vi "CS_Write_Config.vi"(4 "error in (no error)":errorcluster, 7 "Config refnum":T1) -> (0 "error out":errorcluster, 3 "refnum out":T1)   [LabVIEW 2015]
uses:
  <vilib>/Utility/config.llb/Config Data RefNum.ctl
  GSP_Wavelength_Global.vi
  <vilib>/Utility/config.llb/Write Key (Double).vi
  <vilib>/Utility/config.llb/NI_LVConfig.lvlib
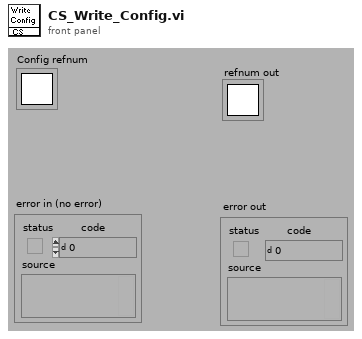
[diagram p1: front panel]
types:
  T1 = typedef "NI_LVConfig.lvlib/Config Data RefNum.ctl" = refnum<k1>
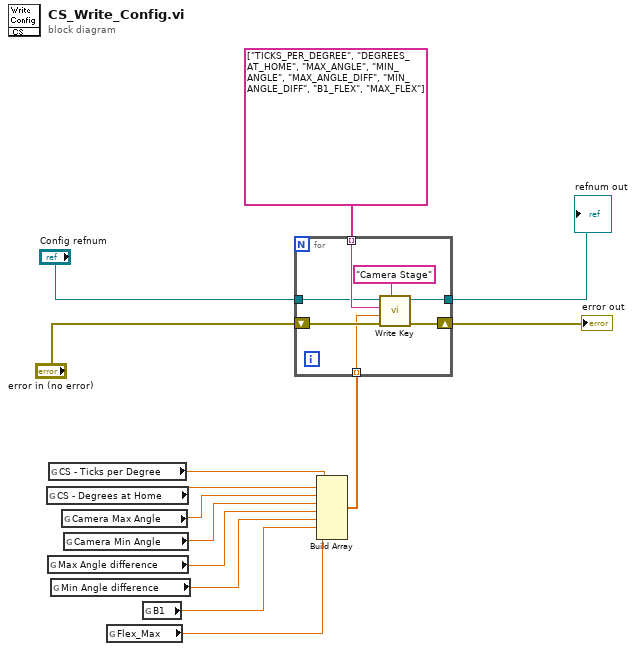
[diagram p0: block diagram]
diagram:
  n1 = global read "GSP_Wavelength_Global.vi" "CS - Degrees at Home"() -> (w13:dbl)
  n2 = global read "GSP_Wavelength_Global.vi" "Max Angle difference"() -> (w4:dbl)
  n3 = global read "GSP_Wavelength_Global.vi" "CS - Ticks per Degree"() -> (w14:dbl)
  n4 = global read "GSP_Wavelength_Global.vi" "Min Angle difference"() -> (w3:dbl)
  n5 = global read "GSP_Wavelength_Global.vi" "Camera Max Angle"() -> (w6:dbl)
  n6 = global read "GSP_Wavelength_Global.vi" "Camera Min Angle"() -> (w5:dbl)
  n7 = global read "GSP_Wavelength_Global.vi" "Flex_Max"() -> (w1:dbl)
  n8 = global read "GSP_Wavelength_Global.vi" "B1"() -> (w2:dbl)
  n9 = Build Array(w14, w13, w6, w5, w4, w3, w2, w1) -> (w12:dbl[])
  n10 = for {
    shift-right: [w19] -> w10
    shift-left: "error in (no error)" -> [w21]
    tunnel: [w18] -> w9
    tunnel: w12 -> [w17] mode=indexing
    tunnel: string[] ["TICKS_PER_DEGREE", "DEGREES_AT_HOME", "MAX_ANGLE", "MIN_ANGLE", "MAX_ANGLE_DIFF", "MIN_ANGLE_DIFF", "B1_FLEX", "MAX_FLEX"] -> [w16] mode=indexing
    tunnel: "Config refnum" -> [w15]
    n11 = call-poly <vilib>:"Write Key.vi"("section"="Camera Stage", "error in (no error)"=w21, "value"=w17, "key"=w16, "refnum"=w15) -> ("error out"=w19:errorcluster, "refnum out"=w18:T1)  [unwired: 4 in, 1 out]
  }
  "error out" <- w10
  "refnum out" <- w9
